vi "Property Tree Symbol & Indent.vi"(7 "Action":T1, 10 "Tree Type":enum16{"Main", "Write", "Read"}(ring), 11 "Property Info":T2) -> (1 "Child Only?":bool, 2 "Indent":u16, 3 "Symbol":i32=38)   [LabVIEW 2023]
uses:
  controls/action enum.ctl
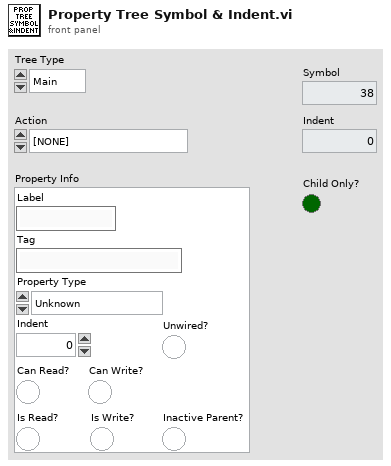
[diagram p1: front panel]
types:
  T1 = typedef "action enum.ctl" = enum16{"[NONE]", "Wire Bundle", "Wire Unbundle", "Terminal Unbundle", "Terminal Bundle", "Bundler Move Up", "Bundler Move Down", "Bundler Insert", "Bundler Remove", "Bundler Remove Unwired", "Bundler Rearrange", "In Place Insert", "In Place Remove", "In Place Remove Unwired", "In Place Rearrange", "Wire Properties", "Wire Method", "Terminal Properties", "Terminal Method", "Property Move Up", "Property Move Down", "Properties Insert", "Properties Remove", "Properties Remove Unwired", "Properties Rearrange", "Method Change", "Class for Constant", "Class For Control", "Class For Node", "Class Name to Clipboard"}
  T2 = cluster{"Label":string, "Tag":string, "Property Type":enum16{"Unknown", "Base", "Scripting", "Private", "Deprecated", "None", "Divider"}, "Indent":u16, "Can Read?":bool, "Can Write?":bool, "Is Read?":bool, "Is Write?":bool, "Inactive Parent?":bool, "Unwired?":bool}
  T3 = enum16{"Unknown", "Base", "Scripting", "Private", "Deprecated", "None", "Divider"}
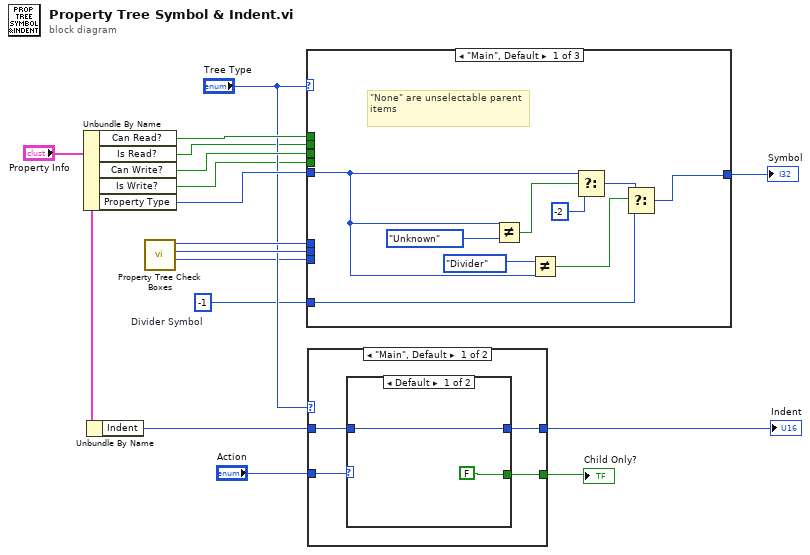
[diagram p0: block diagram]
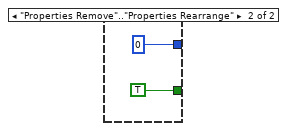
[diagram p2: hidden frame]
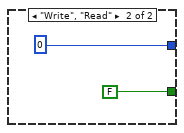
[diagram p3: hidden frame]
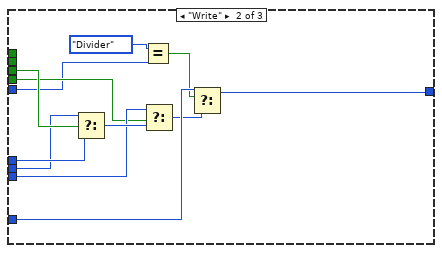
[diagram p4: hidden frame]
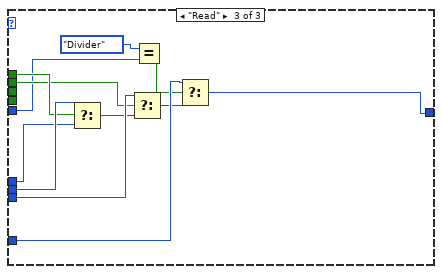
[diagram p5: hidden frame]
diagram:
  w6 = -1  # Divider Symbol
  n1 = Unbundle By Name("Property Info") -> ("Can Read?"=w13:bool, "Is Read?"=w8:bool, "Can Write?"=w16:bool, "Is Write?"=w7:bool, "Property Type"=w15:T3)
  n2 = Unbundle By Name("Property Info") -> ("Indent"=w14:u16)
  n3 = call "Property Tree Check Boxes.vi"() -> ("Checked"=w5:i32, "Unchecked"=w12:i32, "None"=w11:i32)  [unwired: 9 in]
  n4 = case shown="\"Main\", Default" "Tree Type" {
    tunnel: w11 -> [_ w36 w48]
    tunnel: w16 -> [_ w37 _]
    tunnel: [w18 w29 w41] -> w4
    tunnel: w15 -> [w17 w27 w39]
    tunnel: w12 -> [_ w35 w49]
    tunnel: w13 -> [_ _ w47]
    tunnel: w5 -> [_ w33 w46]
    tunnel: w8 -> [_ _ w45]
    tunnel: w7 -> [_ w32 _]
    tunnel: w6 -> [w20 w31 w43]
    frame "Main", Default {
      # "\"None\" are unselectable parent items"
      n5 = Not Equal?(x=w17, y=T3."Unknown" ("Property Type")) -> (x != y?=w25:bool)
      n6 = Not Equal?(x=T3."Divider" ("Property Type"), y=w17) -> (x != y?=w21:bool)
      n7 = Select(t=w17, s=w25, f=-2) -> (s? t:f=w19:i32)
      n8 = Select(t=w19, s=w21, f=w20) -> (s? t:f=w18:i32)
    }
    frame "Write" {
      n9 = Select(t=w35, s=w37, f=w36) -> (s? t:f=w34:i32)
      n10 = Equal?(x=T3."Divider" ("Property Type"), y=w27) -> (x = y?=w26:bool)
      n11 = Select(t=w33, s=w32, f=w34) -> (s? t:f=w30:i32)
      n12 = Select(t=w31, s=w26, f=w30) -> (s? t:f=w29:i32)
    }
    frame "Read" {
      n13 = Select(t=w49, s=w47, f=w48) -> (s? t:f=w44:i32)
      n14 = Select(t=w46, s=w45, f=w44) -> (s? t:f=w42:i32)
      n15 = Equal?(x=T3."Divider" ("Property Type"), y=w39) -> (x = y?=w38:bool)
      n16 = Select(t=w43, s=w38, f=w42) -> (s? t:f=w41:i32)
    }
  }
  "Symbol" <- w4
  n17 = case shown="\"Main\", Default" "Tree Type" {
    tunnel: w14 -> [w51 _]
    tunnel: [w52 0] -> w3
    tunnel: "Action" -> [w53 _]
    tunnel: [w50 FALSE] -> w1
    frame "Main", Default {
      n18 = case shown="Default" w53 {
        tunnel: [w55 0] -> w52
        tunnel: w51 -> [w55 _]
        tunnel: [FALSE TRUE] -> w50
        frame Default {
        }
        frame "Properties Remove".."Properties Rearrange" {
        }
      }
    }
    frame "Write", "Read" {
    }
  }
  "Indent" <- w3
  "Child Only?" <- w1
